vi "Rele_resistencia.vi"() -> ()   [LabVIEW 2018]
uses:
  <vilib>/Platform/TimedLoop/XDataNode/timing_clust.ctl
  <vilib>/Platform/TimedLoop/XDataNode/nitl_modes.ctl
  <vilib>/Platform/TimedLoop/XDataNode/wakeup.ctl
  <vilib>/DAQmx/write.llb/DAQmx Write (Counter Frequency 1Chan 1Samp).vi
  <vilib>/DAQmx/create/channels.llb/DAQmx Create Channel (CO-Pulse Generation-Frequency).vi
  <vilib>/DAQmx/configure/timing.llb/DAQmx Timing (Implicit).vi
  <vilib>/DAQmx/miscellaneous.llb/DAQmx Fill In Error Info.vi
  <vilib>/platform/TimedLoop/XDataNode/XDataNode.xnode
  <resource>/objmgr/daqmx.rc
  <vilib>/Platform/TimedLoop/XDataNode/XDNodeRunTimeDep.lvlib
panel:
  out "Temperatura Res. Intermed":cluster{dbl[], dbl[]}(graph)
  out "D.C. Res. Intermed":cluster{dbl[], dbl[]}(graph)
  out "D.C. Res. Descarga":cluster{dbl[], dbl[]}(graph)
  in  "duty cycle intermed":dbl=1.19209297e-07 min=1.19209297e-07 max=0.999999881
  out "Temperatura Reservatorio Descarga":cluster{dbl[], dbl[]}(graph)
  out "error out":errorcluster
  in  "duty cycle descarga":dbl=1.19209297e-07 min=1.19209297e-07 max=0.999999881
  in  "STOP":bool
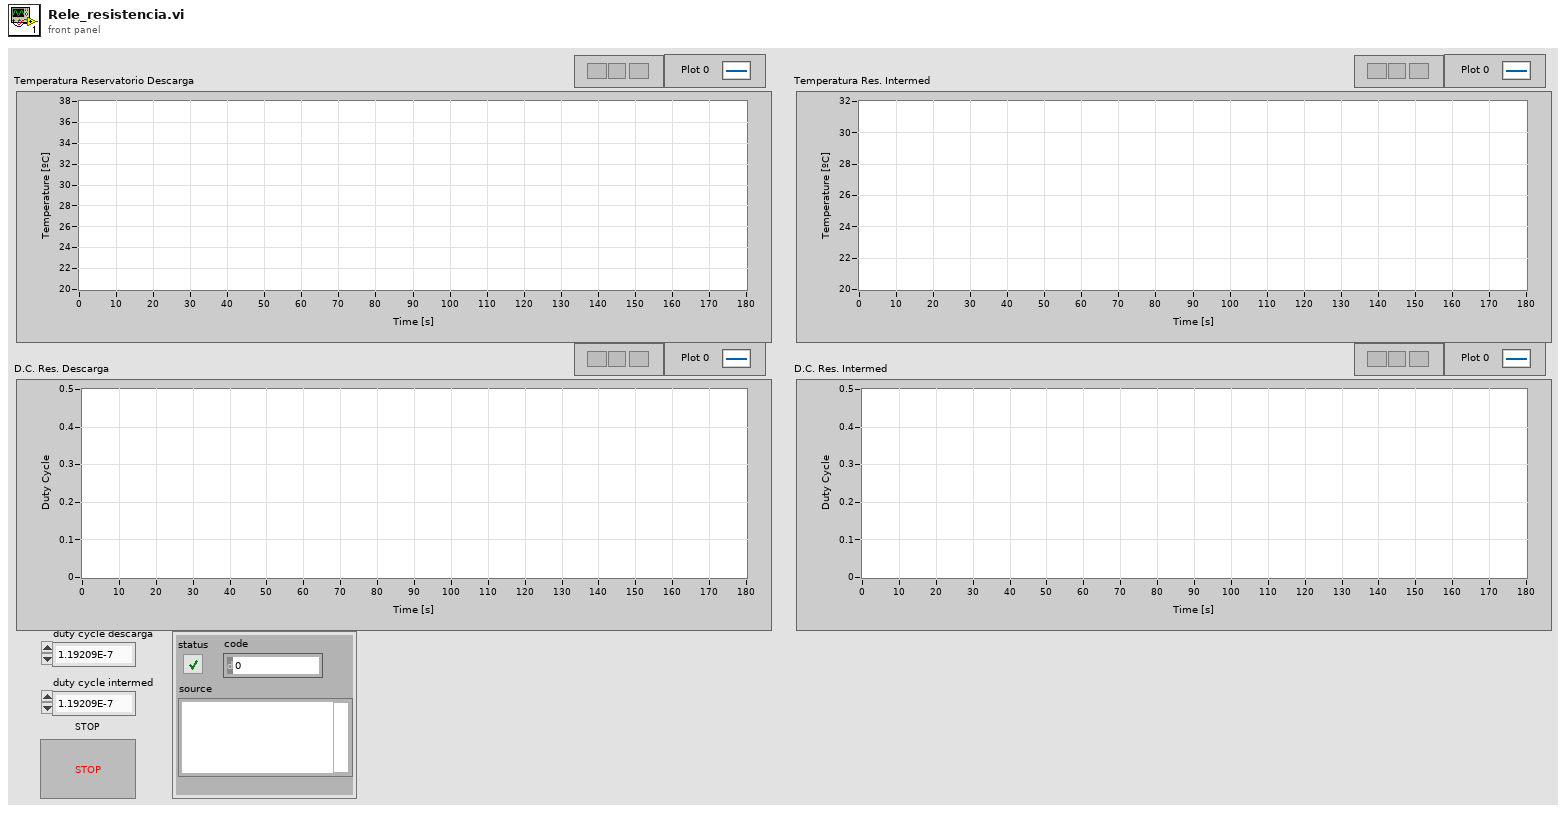
[diagram p1: front panel]
types:
  T1 = typedef "XDNodeRunTimeDep.lvlib/timing_clust.ctl" = cluster{"Expected End [f-1]":u64, "Actual End [f-1]":u64, "Finished Late? [f-1]":bool, "Expected End [i-1]":u64, "Actual End [i-1]":u64, "Finished Late? [i-1]":bool, "Expected Start [i]":u64, "Actual Start [i]":u64, "Expected Start [f]":u64, "Actual Start [f]":u64, "Source Name":string, "Structure Name":string, "Period":i64, "Deadline":i64, "Offset":i64, "Start":i64, "Priority":i32, "Timeout":i32, "Mode":T2, "Wakeup Reason":T3, "Error":errorcluster, "Source Type":string, "Secondary Source Type":string, "Global End Time":u64, "Global Start Time":u64, "Frame Duration":u64, "Iteration Duration":u64, "Assigned CPU":i32, "I/O Scan Engine Mode":u32}
  T2 = typedef "XDNodeRunTimeDep.lvlib/nitl_modes.ctl" = enum32{"No Change", "Process missed periods, maintain original phase", "Discard missed periods, maintain original phase", "Process missed periods, ignore original phase", "Discard missed periods, ignore original phase"}
  T3 = typedef "XDNodeRunTimeDep.lvlib/wakeup.ctl" = enum32{"Normal", "Aborted", "Asynchronous wakeup", "Timing source error", "Timed loop error", "Timeout"}
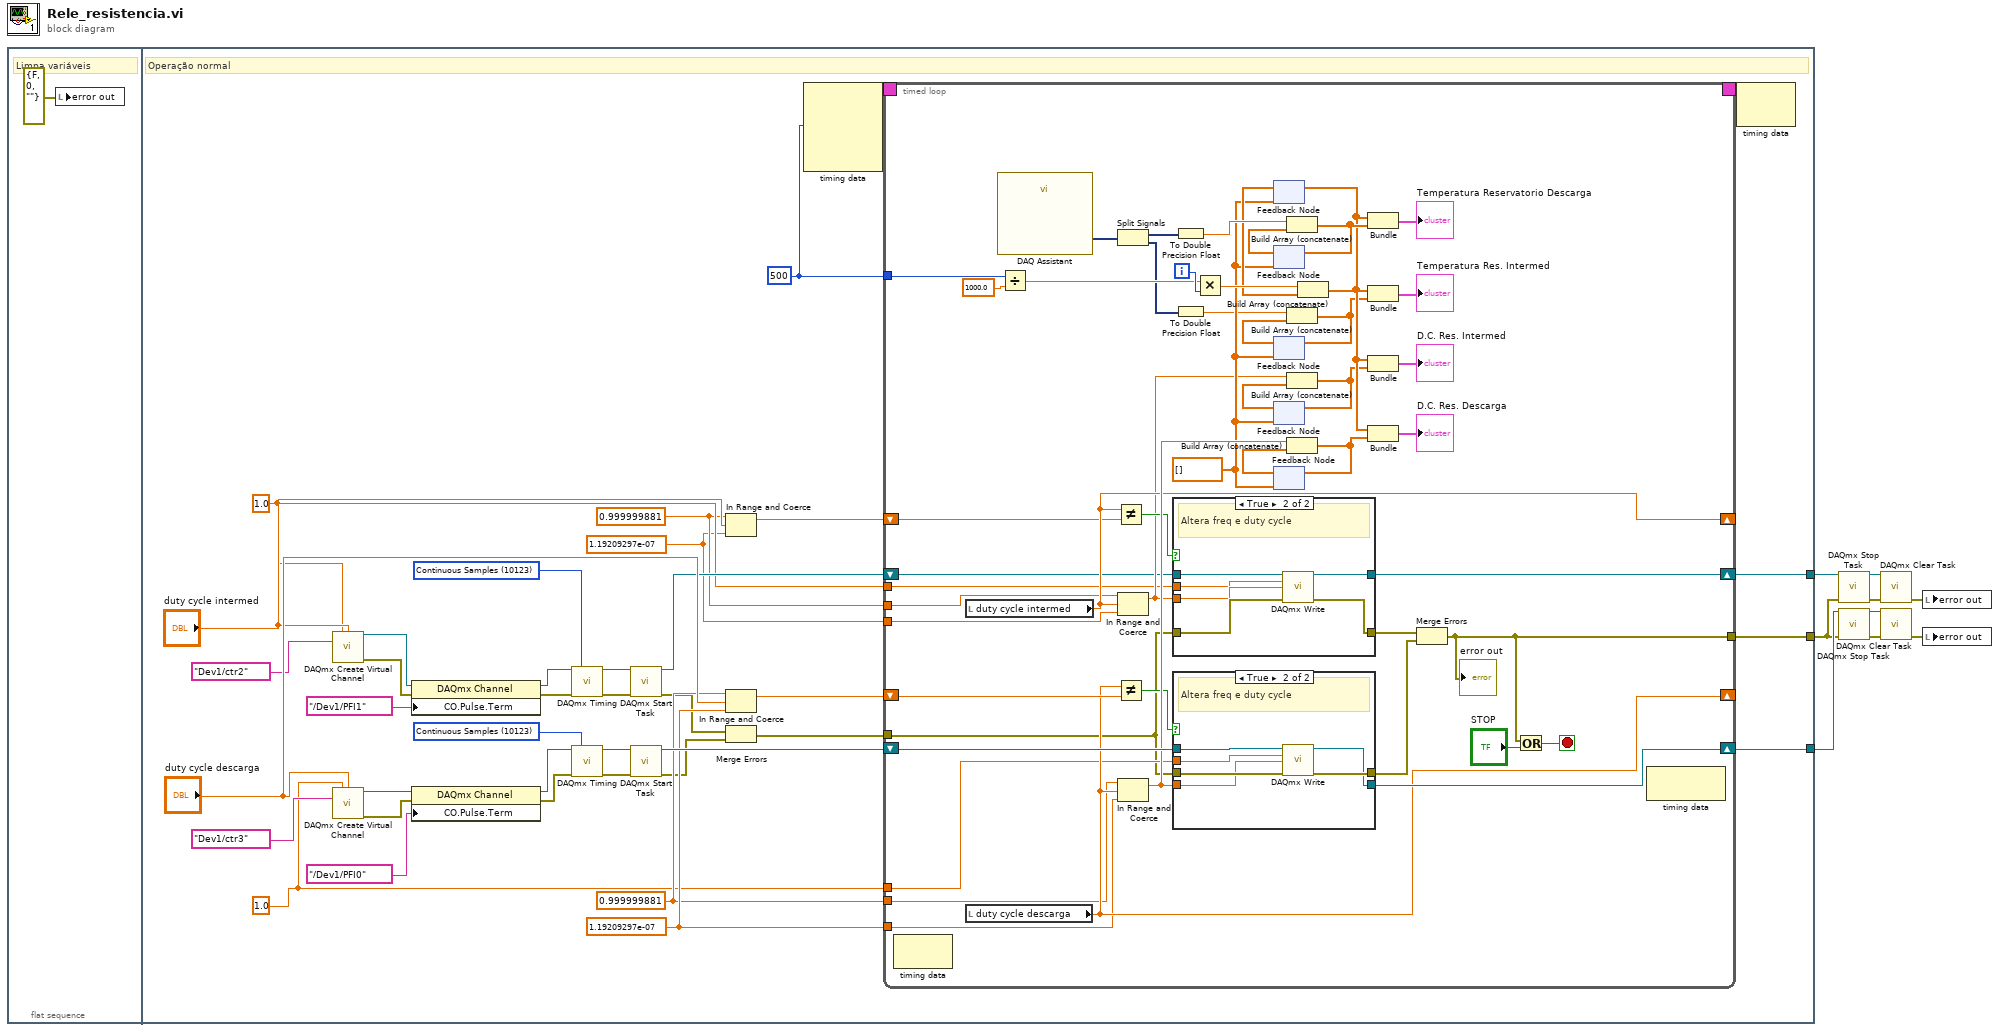
[diagram p0: block diagram]
diagram:
  n1 = flat-sequence {
    tunnel: [w34] -> w6
    tunnel: [w35] -> w2
    tunnel: [w11] -> w1
    frame #0 {
      # "Limpa variáveis"
      n2 = local write "error out"(errorcluster {"status"=FALSE, "code"=0, "source"=""} ("error out")) -> ()
    }
    frame #1 {
      w14 = 1.0 ("frequency")
      w12 = 1.19209297e-07 ("lower limit")
      w13 = 0.999999881 ("lower limit")
      w27 = 10123 items=["Finite Samples"=10178, "Continuous Samples"=10123, "Hardware Timed Single Point"=12522] ("sample mode")
      w30 = 1.0 ("frequency")
      w31 = i64 500 ("Period")
      w40 = 1.19209297e-07 ("lower limit")
      w36 = 0.999999881 ("lower limit")
      w39 = 10123 items=["Finite Samples"=10178, "Continuous Samples"=10123, "Hardware Timed Single Point"=12522] ("sample mode")
      # "Operação normal"
      n3 = call-poly <vilib>:"DAQmx Create Virtual Channel.vi"("frequency"=w14, "duty cycle"="duty cycle intermed", "counter"=tag "Dev1/ctr2") -> ("task out"=w26:refnum<k21>, "error out"=w24:errorcluster)  [unwired: 11 in]
      n4 = call-poly <vilib>:"DAQmx Create Virtual Channel.vi"("frequency"=w30, "duty cycle"="duty cycle descarga", "counter"=tag "Dev1/ctr3") -> ("task out"=w42:refnum<k21>, "error out"=w44:errorcluster)  [unwired: 11 in]
      n5 = property class="DAQmx Channel"(reference=w26, error in=w24, "CO.Pulse.Term"=tag "/Dev1/PFI1") -> (reference out=w22:refnum<k21>, error out=w23:errorcluster)
      n6 = property class="DAQmx Channel"(reference=w42, error in=w44, "CO.Pulse.Term"=tag "/Dev1/PFI0") -> (reference out=w46:refnum<k21>, error out=w45:errorcluster)
      n7 = call-poly <vilib>:"DAQmx Timing.vi"("task/channels in"=w22, "sample mode"=w27, "error in"=w23) -> ("task out"=w21:refnum<k21>, "error out"=w25:errorcluster)  [unwired: 11 in]
      n8 = call-poly <vilib>:"DAQmx Timing.vi"("task/channels in"=w46, "sample mode"=w39, "error in"=w45) -> ("task out"=w47:refnum<k21>, "error out"=w43:errorcluster)  [unwired: 11 in]
      n9 = call <vilib>:"DAQmx Start Task.vi"("task/channels in"=w21, "error in"=w25) -> ("task out"=w15:refnum<k21>, "error out"=w17:errorcluster)  [unwired: 12 in]
      n10 = call <vilib>:"DAQmx Start Task.vi"("task/channels in"=w47, "error in"=w43) -> ("task out"=w41:refnum<k21>, "error out"=w18:errorcluster)  [unwired: 12 in]
      n11 = In Range and Coerce(upper limit=w13, x="duty cycle intermed", lower limit=w12) -> (coerced(x)=w16:dbl)  [unwired: 1 out]
      n12 = In Range and Coerce(upper limit=w36, x="duty cycle descarga", lower limit=w40) -> (coerced(x)=w49:dbl)  [unwired: 1 out]
      n13 = Merge Errors(w17, w18) -> (w19:errorcluster)
      n14 = node-c288(w31) -> (w33:T1)  [unwired: 3 in]
      n15 = timed-loop {
        tunnel: w19 -> [w65]
        tunnel: [w63] -> w35
        shift-right: [w95] -> _
        shift-left: w49 -> [w96]
        tunnel: w36 -> [w94]
        tunnel: w40 -> [w92]
        timing: w33 -> [_]
        timing-out: [_] -> w32
        tunnel: w31 -> [w90]
        tunnel: w30 -> [w83]
        shift-right: [w69] -> _
        shift-left: w16 -> [w66]
        shift-right: [w97] -> w34
        shift-left: w41 -> [w98]
        shift-right: [w60] -> w11
        shift-left: w15 -> [w61]
        tunnel: w14 -> [w59]
        tunnel: w13 -> [w58]
        tunnel: w12 -> [w57]
        i -> [w91]
        stop <- w93 stop-if-true
        w74 = dbl[] []
        n16 = node-c288() -> ()  [unwired: 1 in, 1 out]
        n17 = local read "duty cycle intermed"() -> (w69:dbl)
        n18 = local read "duty cycle descarga"() -> (w95:dbl)
        n19 = call "DAQ Assistant"() -> ("data"=w56:dynamicdata)  [unwired: 17 in, 2 out]
        n20 = Divide(x=w90, y=1000.0) -> (x/y=w85:dbl)
        n21 = Not Equal?(x=w69, y=w66) -> (x != y?=w70:bool)
        n22 = Not Equal?(x=w95, y=w96) -> (x != y?=w71:bool)
        n23 = Split Signals(w56) -> (w55:dynamicdata, w54:dynamicdata)  [unwired: 2 in]
        n24 = In Range and Coerce(upper limit=w58, x=w69, lower limit=w57) -> (coerced(x)=w68:dbl)  [unwired: 1 out]
        n25 = In Range and Coerce(upper limit=w94, x=w95, lower limit=w92) -> (coerced(x)=w87:dbl)  [unwired: 1 out]
        n26 = case shown="True" w70 {
          tunnel: w65 -> [w99 w106]
          tunnel: [w99 w105] -> w62
          tunnel: [w100 w104] -> w60
          tunnel: w61 -> [w100 w103]
          tunnel: w68 -> [_ w102]
          tunnel: w59 -> [_ w101]
          frame False {
          }
          frame True {
            # "Altera freq e duty cycle"
            n27 = call-poly <vilib>:"DAQmx Write.vi"("task/channels in"=w103, "frequency"=w101, "duty cycle"=w102, "error in"=w106) -> ("task out"=w104:refnum<k21>, "error out"=w105:errorcluster)  [unwired: 9 in, 1 out]
          }
        }
        n28 = case shown="True" w71 {
          tunnel: w65 -> [w107 w114]
          tunnel: [w107 w113] -> w64
          tunnel: [w108 w112] -> w97
          tunnel: w98 -> [w108 w111]
          tunnel: w87 -> [_ w110]
          tunnel: w83 -> [_ w109]
          frame False {
          }
          frame True {
            # "Altera freq e duty cycle"
            n29 = call-poly <vilib>:"DAQmx Write.vi"("task/channels in"=w111, "frequency"=w109, "duty cycle"=w110, "error in"=w114) -> ("task out"=w112:refnum<k21>, "error out"=w113:errorcluster)  [unwired: 9 in, 1 out]
          }
        }
        n30 = To Double Precision Float(number=w55) -> (double precision float=w88:dbl)
        n31 = To Double Precision Float(number=w54) -> (double precision float=w52:dbl)
        n32 = Multiply(x=w85, y=w91) -> (x*y=w84:dbl)
        n33 = feedback #1(w74) -> (w78:dbl[])
        n34 = feedback #2(w74) -> (w79:dbl[])
        n35 = feedback #3(w74) -> (w73:dbl[])
        n36 = feedback #4(w74) -> (w75:dbl[])
        n37 = feedback #5(w74) -> (w76:dbl[])
        n38 = Build Array (concatenate)(w88, w79) -> (w80:dbl[])
        n39 = feedback-in #2(w80) -> ()
        n40 = Build Array (concatenate)(w52, w73) -> (w50:dbl[])
        n41 = feedback-in #3(w50) -> ()
        n42 = Build Array (concatenate)(w68, w75) -> (w51:dbl[])
        n43 = feedback-in #4(w51) -> ()
        n44 = Build Array (concatenate)(w87, w76) -> (w77:dbl[])
        n45 = feedback-in #5(w77) -> ()
        n46 = Build Array (concatenate)(w84, w78) -> (w72:dbl[])
        n47 = feedback-in #1(w72) -> ()
        n48 = Bundle(w72, w80) -> (→"Temperatura Reservatorio Descarga":cluster{dbl[], dbl[]})  [unwired: 1 in]
        n49 = Bundle(w72, w50) -> (→"Temperatura Res. Intermed":cluster{dbl[], dbl[]})  [unwired: 1 in]
        n50 = Bundle(w72, w51) -> (→"D.C. Res. Intermed":cluster{dbl[], dbl[]})  [unwired: 1 in]
        n51 = Bundle(w72, w77) -> (→"D.C. Res. Descarga":cluster{dbl[], dbl[]})  [unwired: 1 in]
        n52 = Merge Errors(w62, w64) -> (w63:errorcluster)
        "error out" <- w63
        n53 = Or(x=w63, y="STOP") -> (x .or. y?=w93:bool)
        n54 = node-c288() -> ()  [unwired: 1 in, 1 out]
      }
      n55 = node-c288(w32) -> ()  [unwired: 1 out]
    }
  }
  n56 = call <vilib>:"DAQmx Stop Task.vi"("task/channels in"=w1, "error in"=w2) -> ("task out"=w4:refnum<k21>, "error out"=w3:errorcluster)  [unwired: 12 in]
  n57 = call <vilib>:"DAQmx Stop Task.vi"("task/channels in"=w6, "error in"=w2) -> ("task out"=w8:refnum<k21>, "error out"=w9:errorcluster)  [unwired: 12 in]
  n58 = call <vilib>:"DAQmx Clear Task.vi"("task in"=w4, "error in"=w3) -> ("error out"=w5:errorcluster)  [unwired: 13 in]
  n59 = call <vilib>:"DAQmx Clear Task.vi"("task in"=w8, "error in"=w9) -> ("error out"=w7:errorcluster)  [unwired: 13 in]
  n60 = local write "error out"(w5) -> ()
  n61 = local write "error out"(w7) -> ()
